vi "Roboteq_MDC_motor_control.vi"() -> ()   [LabVIEW 2019]
uses:
  <vilib>/myRIO/Instrument Drivers/Onboard IO/UART/typedef/VISA Configuration.ctl
  <vilib>/Instr/_visa.llb/VISA Configure Serial Port (Instr).vi
  <vilib>/FPGAPlugInAG/myRIO-1900/niLvFpga_Open_myRIO-1900.vi
  <vilib>/rvi/interface/common/dynamic/niFpgaDynamicAddResources.vi
  <vilib>/Utility/error.llb/Error Cluster From Error Code.vi
  <vilib>/rvi/errors/niLvFpgaAdjustHostInterfaceError.vi
  <vilib>/FPGAPlugInAG/Dynamic/niLvFpga_Close_Dynamic.vi
  <vilib>/rvi/interface/nirviOpenFPGA/nirviOpenFPGA.xnode
  FPGA Bitfiles/robotproject_FPGATarget_PulsePeriodMeasu_AqxrhuZqRsc.lvbitx
  Pulse_Period_Measurement.vi
  <vilib>/rvi/interface/nirviReadWriteControl/nirviReadWriteControl.xnode
  <vilib>/rvi/interface/nirviCloseFPGA/nirviCloseFPGA.xnode
  <vilib>/myRIO/Instrument Drivers/Onboard IO/UART/UART.lvlib
  <vilib>/rvi/interface/Simulation/niFpgaSimulationCallBeginRW.vi
  NiFpgaLv.dll
panel:
  out "error out 2":errorcluster
  out "concatenated string 6":string
  out "concatenated string 5":string
  out "concatenated string 4":string
  out "concatenated string 3":string
  out "concatenated string 2":string
  out "concatenated string":string
  in  "VISA resource name":refnum<visa-resource-name>
  in  "error in (no error)":errorcluster
  out "MODE_SWITCH":u32
  out "ON_OFF_SWITCH":u32
  out "R_THROTTLE":u32
  out "L_THROTTLE":u32
  out "L_MOTOR":i32(slide) scale=-500.0..500.0
  out "R_MOTOR":i32(slide) scale=-500.0..500.0
  in  "stop":bool
  out "VISA state":string
  out "On / Off":bool
  out "Mode":bool
  out "State":string
  out "error out":errorcluster
  # "on_manual"
  # "off"
  # "Mode_auto"
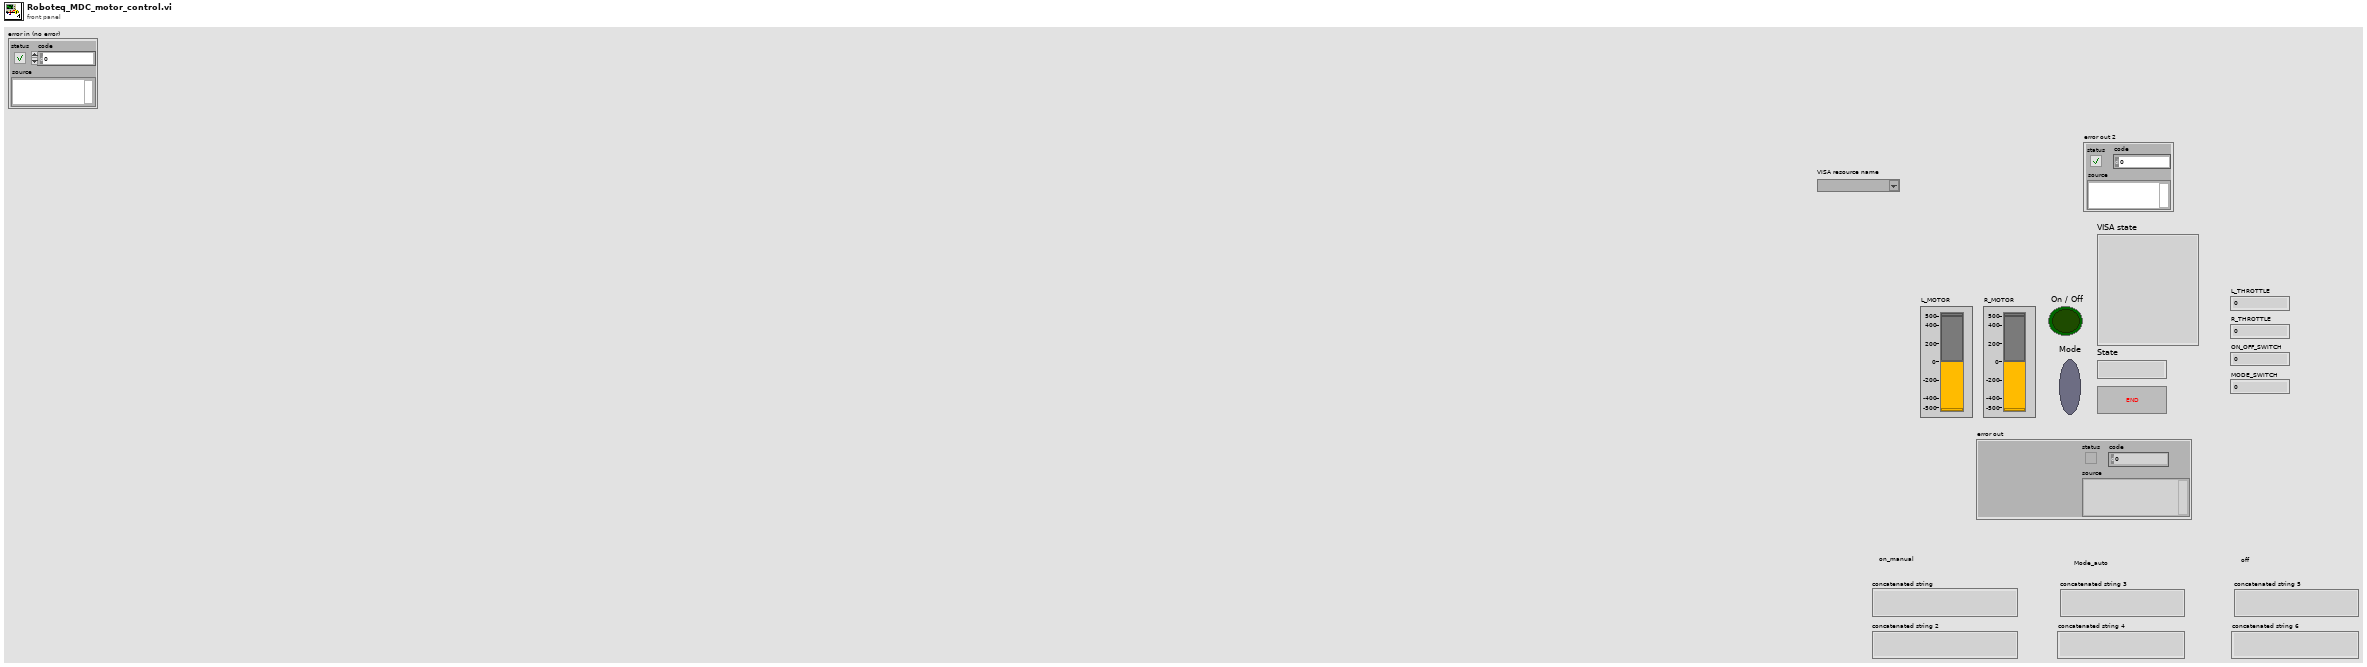
[diagram p1: front panel]
types:
  T1 = typedef "UART.lvlib/VISA Configuration.ctl" = cluster{"baud rate (9600)":u32, "data bits (8)":u16, "parity (0:none)":enum16{"None", "Odd", "Even", "Mark", "Space"}, "stop bits (10: 1 bit)":u16, "flow control (0:none)":u16, "termination char\n(0xA = '\\n' = LF) ":u8, "Enable Termination\nChar (T)":bool, "timeout (10sec)":u32}
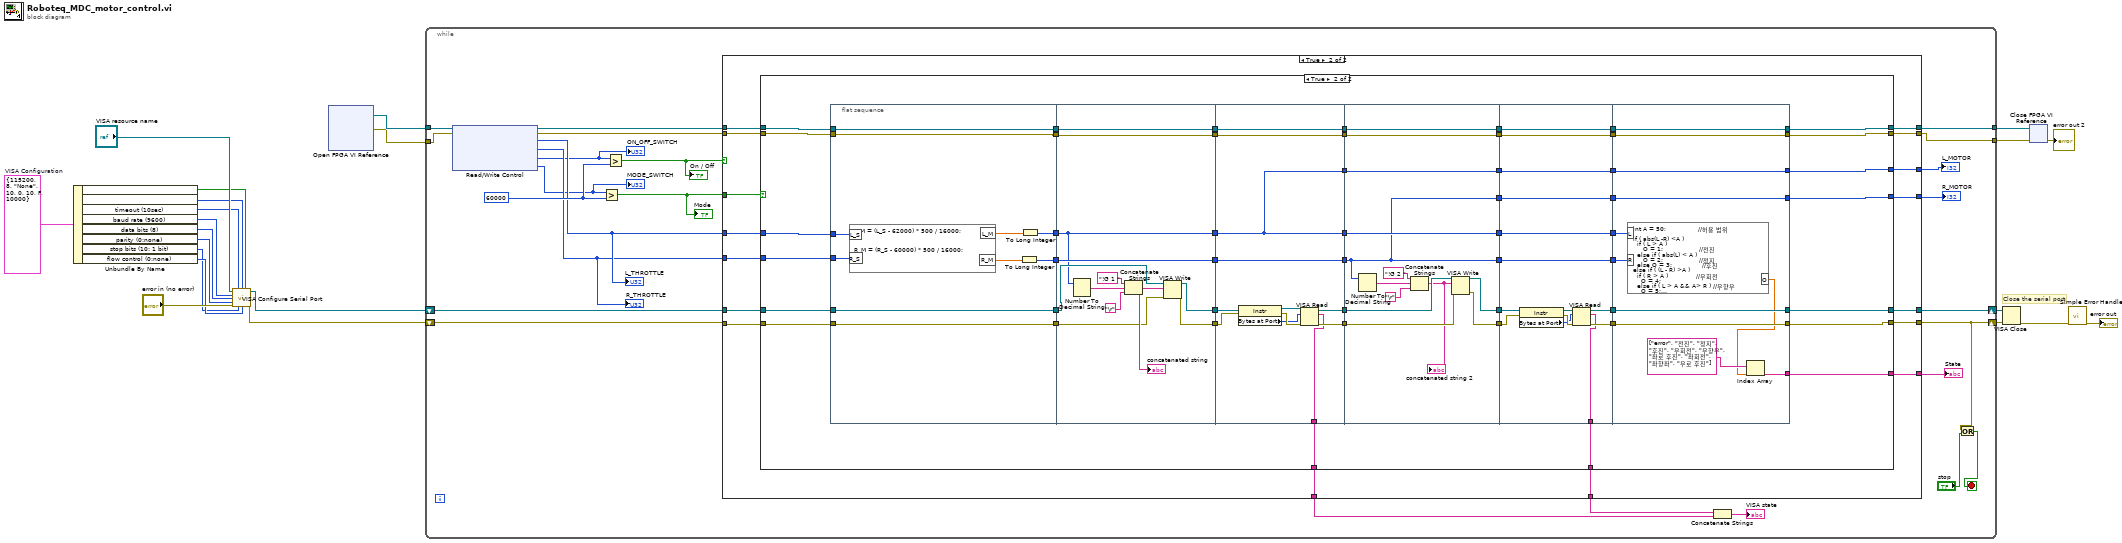
[diagram p0: block diagram]
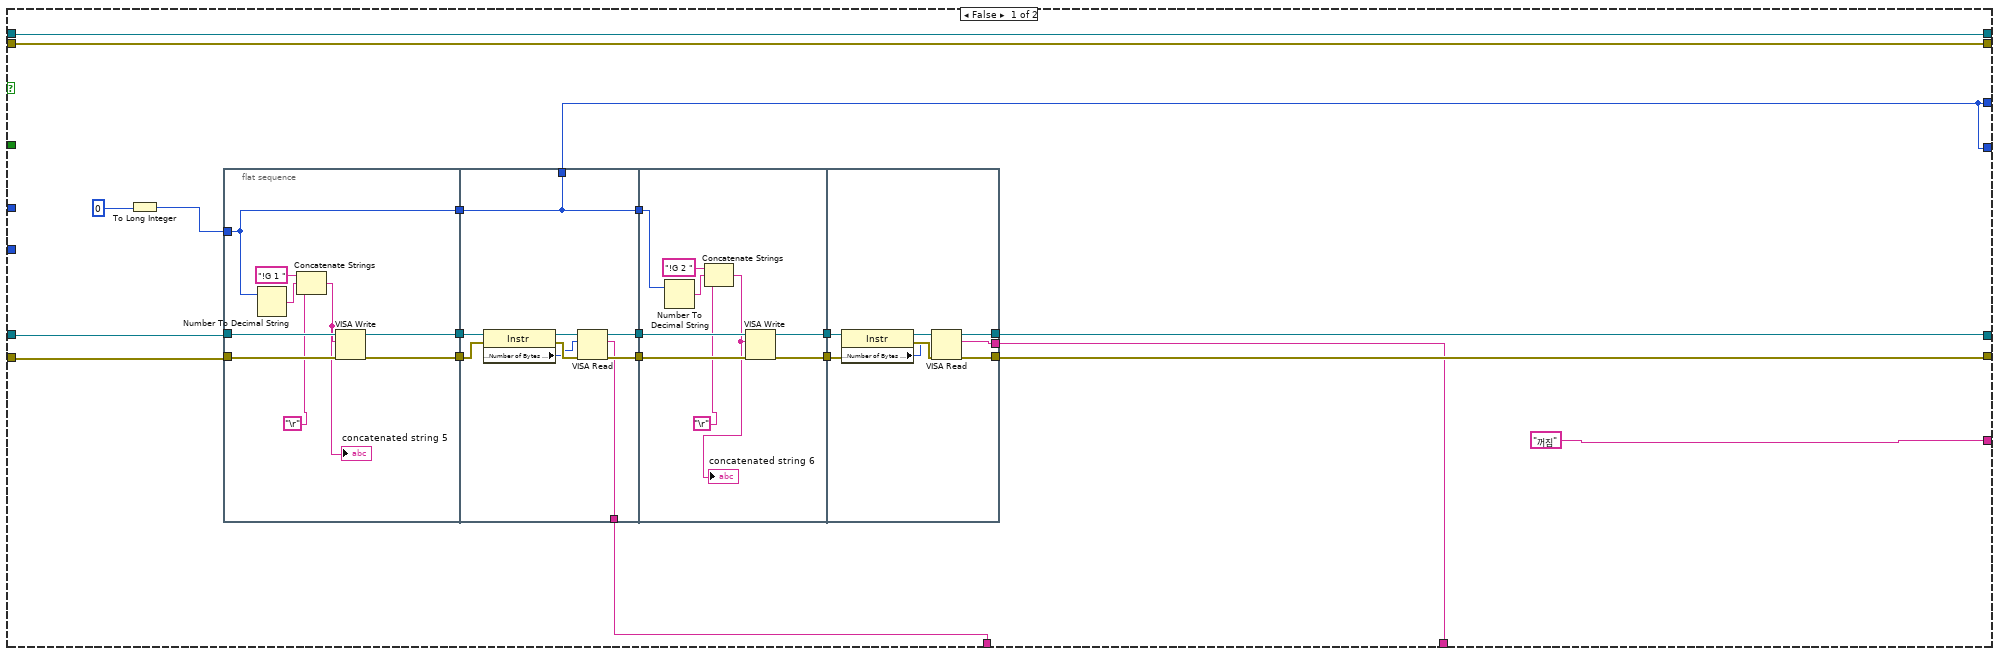
[diagram p2: hidden frame]
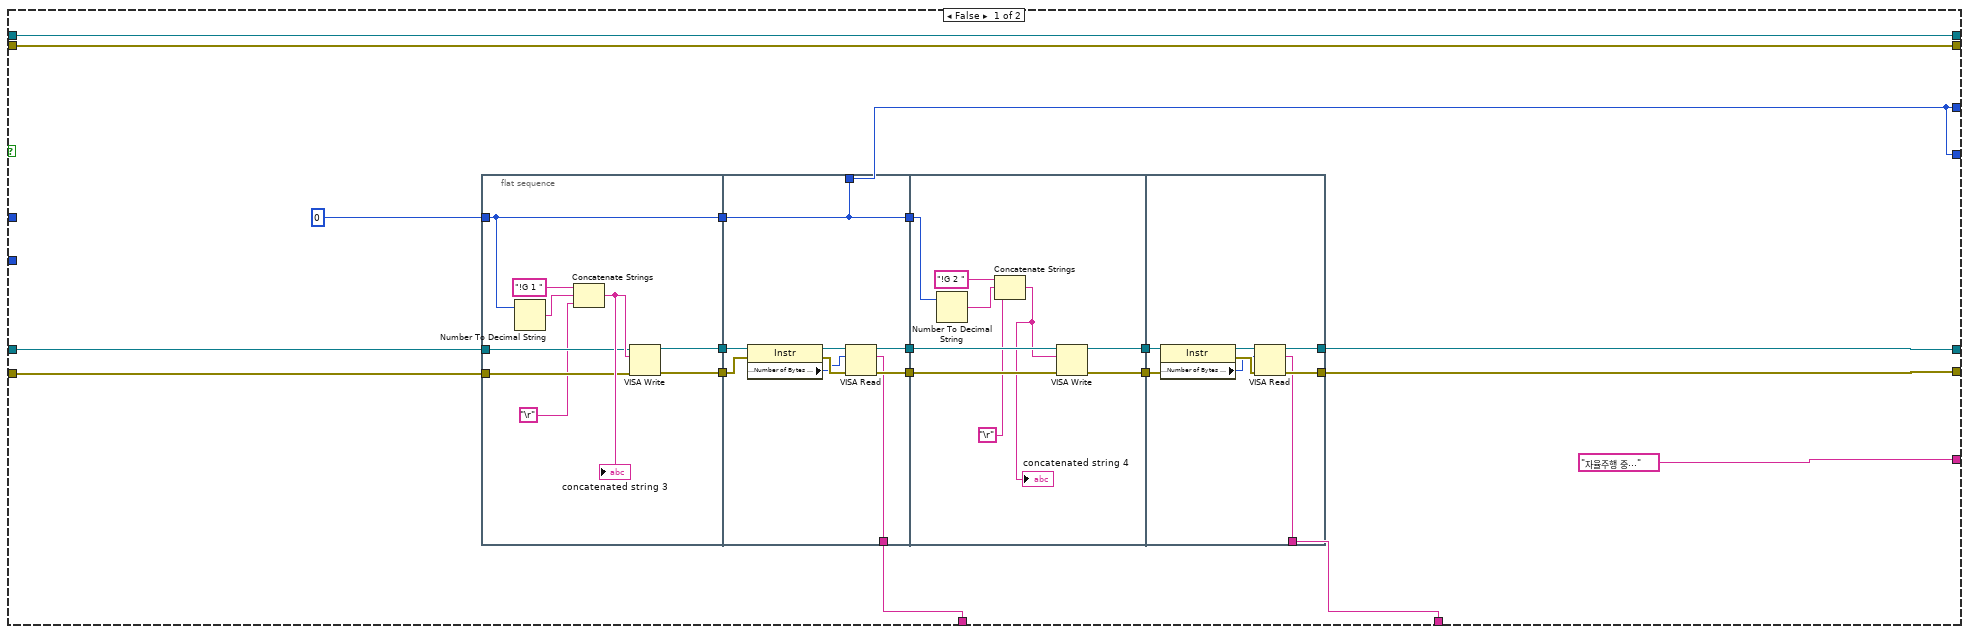
[diagram p3: hidden frame]
diagram:
  w15 = T1 {"baud rate (9600)"=115200, "data bits (8)"=8, "parity (0:none)"=enum."None", "stop bits (10: 1 bit)"=10, "flow control (0:none)"=0, "termination char\n(0xA = '\\n' = LF) "=10, "Enable Termination\nChar (T)"=FALSE, "timeout (10sec)"=10000}  # VISA Configuration
  # "Close the serial port"
  n1 = Unbundle By Name(w15) -> ("Enable Termination\nChar (T)"=w13:bool, "termination char\n(0xA = '\\n' = LF)"=w12:u8, "timeout (10sec)"=w11:u32, "baud rate (9600)"=w6:u32, "data bits (8)"=w7:u16, "parity (0:none)"=w8:enum16{"None", "Odd", "Even", "Mark", "Space"}, "stop bits (10: 1 bit)"=w9:u16, "flow control (0:none)"=w10:u16)
  n2 = call-poly "VISA Configure Serial Port"("VISA resource name"="VISA resource name", "timeout (10sec)"=w11, "termination char\n(0xA = '\\n' = LF)"=w12, "Enable Termination\nChar (T)"=w13, "baud rate (9600)"=w6, "data bits (8)"=w7, "parity (0:none)"=w8, "error in (no error)"="error in (no error)", "stop bits (10: 1 bit)"=w9, "flow control (0:none)"=w10) -> ("VISA resource name out"=w5:refnum<visa-resource-name>, "error out"=w4:errorcluster)  [unwired: 4 in]
  n3 = xnode "Open FPGA VI Reference"() -> ("FPGA VI Reference Out"=w19:refnum<k20>, "error out"=w18:errorcluster)  [unwired: 2 in]
  n4 = while {
    shift-right: [w45] -> w21
    shift-left: w5 -> [w47]
    shift-right: [w24] -> w22
    shift-left: w4 -> [w46]
    tunnel: w19 -> [w43]
    tunnel: w18 -> [w41]
    tunnel: [w39] -> w17
    tunnel: [w38] -> w2
    stop <- w23 stop-if-true
    w37 = u32 60000
    n5 = xnode "Read/Write Control"("FPGA VI Reference In"=w43, "error in"=w41) -> ("FPGA VI Reference Out"=w42:refnum<k20>, "error out"=w40:errorcluster, "DIO0_L_THROTTLE"=w34:u32, "DIO1_R_THROTTLE"=w33:u32, "DIO2_ON_OFF_SWITCH"=w32:u32, "DIO3_MODE_SWITCH"=w31:u32)
    "L_THROTTLE" <- w34
    "R_THROTTLE" <- w33
    "ON_OFF_SWITCH" <- w32
    "MODE_SWITCH" <- w31
    n6 = Greater?(x=w31, y=w37) -> (0:w35:bool)
    "Mode" <- w35
    n7 = Greater?(x=w32, y=w37) -> (0:w36:bool)
    "On / Off" <- w36
    n8 = case shown="True" w36 {
      tunnel: w35 -> [_ w118]
      tunnel: w34 -> [_ w117]
      tunnel: w33 -> [_ w116]
      tunnel: w47 -> [w59 w115]
      tunnel: w46 -> [w58 w114]
      tunnel: [w57 w113] -> w45
      tunnel: [w56 w112] -> w24
      tunnel: ["꺼짐" w111] -> w44
      tunnel: w42 -> [w54 w110]
      tunnel: w40 -> [w53 w109]
      tunnel: [w54 w108] -> w39
      tunnel: [w53 w107] -> w38
      tunnel: [w50 w106] -> w30
      tunnel: [w50 w105] -> w29
      tunnel: [w48 w104] -> w27
      tunnel: [w49 w103] -> w26
      frame False {
        n9 = To Long Integer(number=u32 0) -> (32bit integer=w51:i32)
        n10 = flat-sequence {
          tunnel: [w74] -> w67
          tunnel: [w73] -> w66
          tunnel: w59 -> [w72]
          tunnel: w58 -> [w71]
          tunnel: w51 -> [w70]
          tunnel: [w70] -> w60
          tunnel: [w84] -> w65
          tunnel: w67 -> [w82]
          tunnel: w66 -> [w83]
          tunnel: [w85] -> w64
          tunnel: [w78] -> w61
          tunnel: w60 -> [w78]
          tunnel: [w78] -> w50
          tunnel: [w77] -> w49
          tunnel: w65 -> [w92]
          tunnel: w64 -> [w91]
          tunnel: [w90] -> w63
          tunnel: [w89] -> w62
          tunnel: w61 -> [w88]
          tunnel: w63 -> [w100]
          tunnel: w62 -> [w98]
          tunnel: [w101] -> w56
          tunnel: [w102] -> w57
          tunnel: [w95] -> w48
          frame #0 {
            n11 = Number To Decimal String(number=w70) -> (decimal integer string=w76:string)  [unwired: 1 in]
            n12 = Concatenate Strings("!G 1 " ("string"), w76, "\r") -> (w68:string)
            "concatenated string 5" <- w68
            n13 = VISA Write(VISA resource name=w72, write buffer=w68, error in (no error)=w71) -> (VISA resource name out=w73:refnum<visa-resource-name>, error out=w74:errorcluster)  [unwired: 1 out]
          }
          frame #1 {
            n14 = property class="Instr"(reference=w83, error in=w82) -> (reference out=w79:refnum<visa-resource-name>, error out=w81:errorcluster, "Serial Settings:Number of Bytes at Serial Port"=w80:u32)
            n15 = VISA Read(VISA resource name=w79, byte count=w80, error in (no error)=w81) -> (VISA resource name out=w85:refnum<visa-resource-name>, read buffer=w77:string, error out=w84:errorcluster)  [unwired: 1 out]
          }
          frame #2 {
            n16 = Number To Decimal String(number=w88) -> (decimal integer string=w94:string)  [unwired: 1 in]
            n17 = Concatenate Strings("!G 2 " ("string"), w94, "\r") -> (w86:string)
            "concatenated string 6" <- w86
            n18 = VISA Write(VISA resource name=w91, write buffer=w86, error in (no error)=w92) -> (VISA resource name out=w90:refnum<visa-resource-name>, error out=w89:errorcluster)  [unwired: 1 out]
          }
          frame #3 {
            n19 = property class="Instr"(reference=w100, error in=w98) -> (reference out=w99:refnum<visa-resource-name>, error out=w97:errorcluster, "Serial Settings:Number of Bytes at Serial Port"=w96:u32)
            n20 = VISA Read(VISA resource name=w99, byte count=w96, error in (no error)=w97) -> (VISA resource name out=w102:refnum<visa-resource-name>, read buffer=w95:string, error out=w101:errorcluster)  [unwired: 1 out]
          }
        }
      }
      frame True {
        n21 = case shown="True" w118 {
          tunnel: w117 -> [_ w214]
          tunnel: w116 -> [_ w213]
          tunnel: w115 -> [w127 w201]
          tunnel: w114 -> [w126 w200]
          tunnel: [w125 w199] -> w113
          tunnel: [w124 w198] -> w112
          tunnel: ["자율주행 중..." w197] -> w111
          tunnel: w110 -> [w123 w196]
          tunnel: w109 -> [w122 w195]
          tunnel: [w123 w184] -> w108
          tunnel: [w122 w183] -> w107
          tunnel: [w121 w178] -> w106
          tunnel: [w121 w177] -> w105
          tunnel: [w119 w174] -> w104
          tunnel: [w120 w173] -> w103
          frame False {
            n22 = flat-sequence {
              tunnel: [w143] -> w136
              tunnel: [w142] -> w135
              tunnel: 0 -> [w141]
              tunnel: [w141] -> w134
              tunnel: w127 -> [w140]
              tunnel: w126 -> [w139]
              tunnel: [w154] -> w133
              tunnel: w136 -> [w152]
              tunnel: w135 -> [w153]
              tunnel: [w155] -> w132
              tunnel: [w148] -> w131
              tunnel: w134 -> [w148]
              tunnel: [w148] -> w121
              tunnel: [w147] -> w120
              tunnel: w133 -> [w162]
              tunnel: w132 -> [w161]
              tunnel: [w160] -> w130
              tunnel: [w159] -> w129
              tunnel: w131 -> [w158]
              tunnel: w130 -> [w170]
              tunnel: w129 -> [w168]
              tunnel: [w171] -> w124
              tunnel: [w172] -> w125
              tunnel: [w165] -> w119
              frame #0 {
                n23 = Number To Decimal String(number=w141) -> (decimal integer string=w146:string)  [unwired: 1 in]
                n24 = Concatenate Strings("!G 1 " ("string"), w146, "\r") -> (w144:string)
                "concatenated string 3" <- w144
                n25 = VISA Write(VISA resource name=w140, write buffer=w144, error in (no error)=w139) -> (VISA resource name out=w142:refnum<visa-resource-name>, error out=w143:errorcluster)  [unwired: 1 out]
              }
              frame #1 {
                n26 = property class="Instr"(reference=w153, error in=w152) -> (reference out=w149:refnum<visa-resource-name>, error out=w151:errorcluster, "Serial Settings:Number of Bytes at Serial Port"=w150:u32)
                n27 = VISA Read(VISA resource name=w149, byte count=w150, error in (no error)=w151) -> (VISA resource name out=w155:refnum<visa-resource-name>, read buffer=w147:string, error out=w154:errorcluster)  [unwired: 1 out]
              }
              frame #2 {
                n28 = Number To Decimal String(number=w158) -> (decimal integer string=w164:string)  [unwired: 1 in]
                n29 = Concatenate Strings("!G 2 " ("string"), w164, "\r") -> (w156:string)
                "concatenated string 4" <- w156
                n30 = VISA Write(VISA resource name=w161, write buffer=w156, error in (no error)=w162) -> (VISA resource name out=w160:refnum<visa-resource-name>, error out=w159:errorcluster)  [unwired: 1 out]
              }
              frame #3 {
                n31 = property class="Instr"(reference=w170, error in=w168) -> (reference out=w169:refnum<visa-resource-name>, error out=w167:errorcluster, "Serial Settings:Number of Bytes at Serial Port"=w166:u32)
                n32 = VISA Read(VISA resource name=w169, byte count=w166, error in (no error)=w167) -> (VISA resource name out=w172:refnum<visa-resource-name>, read buffer=w165:string, error out=w171:errorcluster)  [unwired: 1 out]
              }
            }
          }
          frame True {
            n33 = flat-sequence {
              tunnel: w200 -> [w231]
              tunnel: w201 -> [w232]
              tunnel: [w232] -> w216
              tunnel: [w231] -> w215
              tunnel: w214 -> [w230]
              tunnel: w213 -> [w229]
              tunnel: [w225] -> w212
              tunnel: [w223] -> w209
              tunnel: w196 -> [w228]
              tunnel: w195 -> [w227]
              tunnel: [w228] -> w190
              tunnel: [w227] -> w185
              tunnel: [w241] -> w222
              tunnel: [w240] -> w221
              tunnel: w216 -> [w239]
              tunnel: w215 -> [w238]
              tunnel: w212 -> [w234]
              tunnel: [w237] -> w210
              tunnel: w209 -> [w237]
              tunnel: [w236] -> w191
              tunnel: w190 -> [w236]
              tunnel: [w235] -> w186
              tunnel: w185 -> [w235]
              tunnel: [w234] -> w179
              tunnel: [w255] -> w220
              tunnel: w222 -> [w248]
              tunnel: w221 -> [w249]
              tunnel: [w256] -> w219
              tunnel: [w254] -> w173
              tunnel: [w253] -> w211
              tunnel: w210 -> [w253]
              tunnel: [w250] -> w204
              tunnel: [w252] -> w192
              tunnel: w191 -> [w252]
              tunnel: [w251] -> w187
              tunnel: w186 -> [w251]
              tunnel: [w250] -> w180
              tunnel: w179 -> [w250]
              tunnel: w220 -> [w267]
              tunnel: w219 -> [w266]
              tunnel: [w265] -> w218
              tunnel: [w264] -> w217
              tunnel: w211 -> [w259]
              tunnel: [w263] -> w205
              tunnel: w204 -> [w263]
              tunnel: [w259] -> w202
              tunnel: [w262] -> w193
              tunnel: w192 -> [w262]
              tunnel: [w261] -> w188
              tunnel: w187 -> [w261]
              tunnel: [w260] -> w181
              tunnel: w180 -> [w260]
              tunnel: [w259] -> w176
              tunnel: w218 -> [w274]
              tunnel: w217 -> [w273]
              tunnel: [w281] -> w174
              tunnel: [w282] -> w208
              tunnel: [w283] -> w207
              tunnel: [w280] -> w206
              tunnel: w205 -> [w280]
              tunnel: [w279] -> w203
              tunnel: w202 -> [w279]
              tunnel: [w278] -> w194
              tunnel: w193 -> [w278]
              tunnel: [w277] -> w189
              tunnel: w188 -> [w277]
              tunnel: [w276] -> w182
              tunnel: w181 -> [w276]
              tunnel: w176 -> [w275]
              tunnel: [w275] -> w175
              tunnel: [w293] -> w199
              tunnel: [w294] -> w198
              tunnel: w208 -> [w294]
              tunnel: w207 -> [w293]
              tunnel: w206 -> [w292]
              tunnel: w203 -> [w291]
              tunnel: [w288] -> w197
              tunnel: [w287] -> w184
              tunnel: w194 -> [w287]
              tunnel: [w286] -> w183
              tunnel: w189 -> [w286]
              tunnel: w182 -> [w285]
              tunnel: [w285] -> w178
              tunnel: [w284] -> w177
              tunnel: w175 -> [w284]
              frame #0 {
                n34 = formula code="L_M = (L_S - 62000) * 500 / 16000;\n\n\nR_M = (R_S - 60000) * 500 / 16000;"("L_S"=w230, "R_S"=w229) -> ("L_M"=w226:dbl, "R_M"=w224:dbl)
                n35 = To Long Integer(number=w224) -> (32bit integer=w223:i32)
                n36 = To Long Integer(number=w226) -> (32bit integer=w225:i32)
              }
              frame #1 {
                n37 = Number To Decimal String(number=w234) -> (decimal integer string=w244:string)  [unwired: 1 in]
                n38 = Concatenate Strings("!G 1 " ("string"), w244, "\r") -> (w242:string)
                "concatenated string" <- w242
                n39 = VISA Write(VISA resource name=w239, write buffer=w242, error in (no error)=w238) -> (VISA resource name out=w240:refnum<visa-resource-name>, error out=w241:errorcluster)  [unwired: 1 out]
              }
              frame #2 {
                n40 = property class="Instr"(reference=w249, error in=w248) -> (reference out=w247:refnum<visa-resource-name>, error out=w246:errorcluster, "Bytes at Port"=w245:u32)
                n41 = VISA Read(VISA resource name=w247, byte count=w245, error in (no error)=w246) -> (VISA resource name out=w256:refnum<visa-resource-name>, read buffer=w254:string, error out=w255:errorcluster)  [unwired: 1 out]
              }
              frame #3 {
                n42 = Number To Decimal String(number=w259) -> (decimal integer string=w269:string)  [unwired: 1 in]
                n43 = Concatenate Strings("!G 2 " ("string"), w269, "\r") -> (w257:string)
                "concatenated string 2" <- w257
                n44 = VISA Write(VISA resource name=w266, write buffer=w257, error in (no error)=w267) -> (VISA resource name out=w265:refnum<visa-resource-name>, error out=w264:errorcluster)  [unwired: 1 out]
              }
              frame #4 {
                n45 = property class="Instr"(reference=w274, error in=w273) -> (reference out=w272:refnum<visa-resource-name>, error out=w271:errorcluster, "Bytes at Port"=w270:u32)
                n46 = VISA Read(VISA resource name=w272, byte count=w270, error in (no error)=w271) -> (VISA resource name out=w283:refnum<visa-resource-name>, read buffer=w281:string, error out=w282:errorcluster)  [unwired: 1 out]
              }
              frame #5 {
                n47 = formula code="int A = 50;                //허용 범위\n\nif ( abs(L -R) <A )\n  if ( L > A )\n     O = 1;                  //전진\n  else if ( abs(L) < A )\n     O = 2;                  //정지\n  else O = 3;               //후진\nelse if ( (L - R) >A )\n  if ( R > A )              //우회전\n    O = 4;\n  else if ( L > A && A> R ) //우향우\n    O = 5;\n  else O = 6;                 //좌로 후진\nelse \n  if ( L > A )\n    O = 7;                     //좌회전\n  else if ( L < A && A < R )\n    O = 8;                     //좌향좌\n  else O = 9;                 //우로 후진"("L"=w292, "R"=w291) -> ("O"=w289:dbl)
                n48 = Index Array(array=string[] ["error", "전진", "정지", "후진", "우회전", "우향우", "좌로 후진", "좌회전", "좌향좌", "우로 후진"], index=w289) -> (element=w288:string)
              }
            }
          }
        }
      }
    }
    "State" <- w44
    "L_MOTOR" <- w30
    "R_MOTOR" <- w29
    n49 = Concatenate Strings(w27, w26) -> (→"VISA state":string)
    n50 = Or(x=w24, y="stop") -> (x .or. y?=w23:bool)
  }
  n51 = VISA Close(VISA resource name=w21, error in (no error)=w22) -> (error out=w20:errorcluster)
  n52 = xnode "Close FPGA VI Reference"("FPGA VI Reference In"=w17, "error in"=w2) -> ("error out"=→"error out 2":errorcluster)
  n53 = call <vilib>:"Simple Error Handler.vi"("error in (no error)"=w20) -> ("error out"=→"error out":errorcluster)  [unwired: 1 in, 7 out]
